vi "DOE Agilent Setup SUB.vi"(6 "Analog Channels-List":string, 7 "TC Type (K,J,T)":string, 8 "error in (no error)":errorcluster, 9 "TC Channels-List":string, 10 "Agilent Gain":dbl, 11 "VISA Refnum in":refnum<visa-resource-name>) -> (0 "error out":errorcluster, 2 "Clean Analog Scan List":string, 3 "Instrument IDN":string)   [LabVIEW 2016]
uses:
  Drivers/Agilent 34972/Agilent 34970.lvlib
panel:
  out "Total Clean Scan List":string
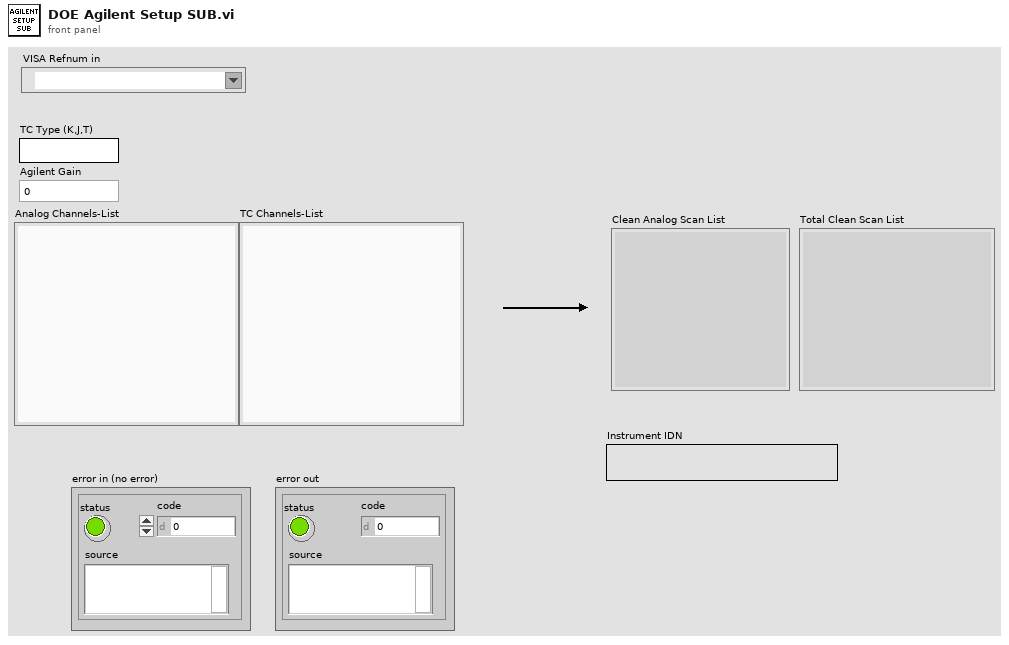
[diagram p1: front panel]
types:
  T1 = cluster{"Timeout Value (10000)":u32, "Baud Rate (57600)":enum16{"1200", "2400", "4800", "9600", "19200", "38400", "57600", "115200"}, "Flow Control (1:XON/XOFF)":enum16{"None", "XON / XOFF", "RTS / CTS", "DTR / DSR"}}
  T2 = enum16{"Thermocouple", "Thermistor", "RTD", "4-Wire RTD"}
  T3 = cluster{"Thermocouple Type (Last)":enum16{"B", "E", "J", "K", "N", "R", "S", "T", "Default (Last)"}, "TC Rjunction (2:Int)":enum16{"Fixed", "External", "Internal"}, "Fixed Rjunction Temp (0:Manual)":enum16{"Manual", "Minimum", "Maximum"}, "TC Auto Check? (F:Don't Check)":bool, "Rjunct Temp Value (0)":dbl}
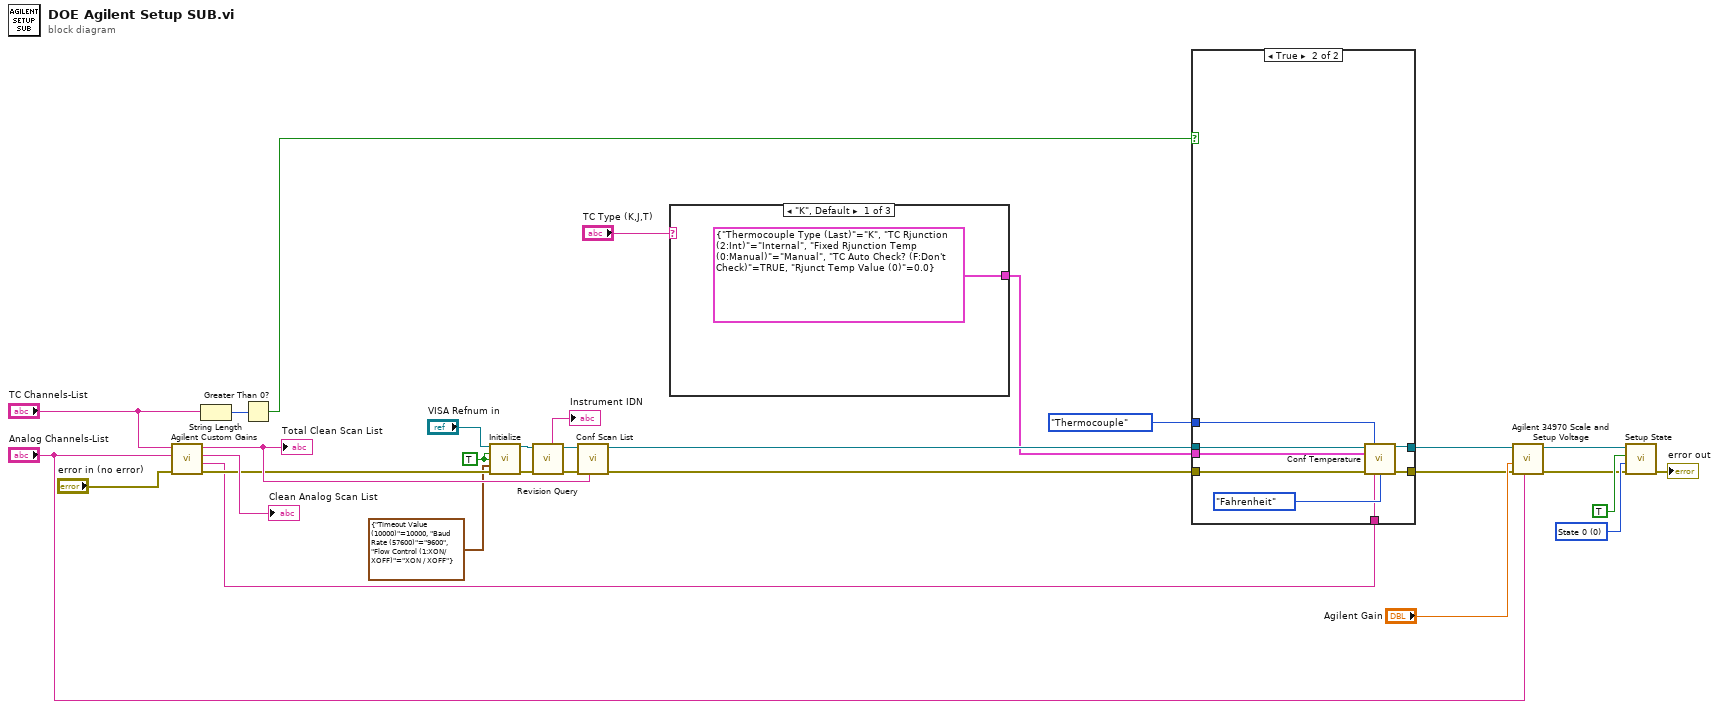
[diagram p0: block diagram]
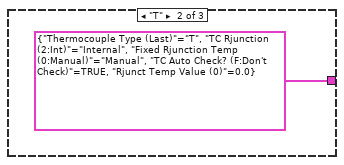
[diagram p3: hidden frame]
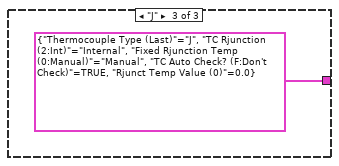
[diagram p4: hidden frame]
diagram:
  w11 = u16 0 items=["State 0", "State 1", "State 2", "State 3", "State 4", "State 5", "Preset State"] ("Setup State (6:Preset)")
  w26 = TRUE ("ID Query (T: Check)")
  n1 = call "Agilent Custom Gains.vi"("Error In"="error in (no error)", "Analog Channels-List"="Analog Channels-List", "TC Channels-List"="TC Channels-List") -> ("Error Out"=w3:errorcluster, "Clean TC Scan List"=w2:string, "Clean Analog Scan List"=→"Clean Analog Scan List":string, "Total Clean Scan List"=w12:string)  [unwired: 5 in]
  "Total Clean Scan List" <- w12
  n2 = String Length(string="TC Channels-List") -> (length=w15:i32)
  n3 = Greater Than 0?(x=w15) -> (x > 0?=w13:bool)
  n4 = call "Initialize.vi"("VISA Resource Name"="VISA Refnum in", "ID Query (T: Check)"=w26, "Reset (T: Reset)"=w26, "Serial Port Configuration"=T1 {"Timeout Value (10000)"=10000, "Baud Rate (57600)"=enum."9600", "Flow Control (1:XON/XOFF)"=enum."XON / XOFF"}, "error in (no error)"=w3) -> ("VISA Resource Name Out"=w25:refnum<visa-resource-name>, "error out"=w24:errorcluster)  [unwired: 9 in]
  n5 = call "Revision Query.vi"("error in (no error)"=w24, "VISA Resource Name"=w25) -> ("error out"=w23:errorcluster, "VISA Resource Name Out"=w22:refnum<visa-resource-name>, "Instrument IDN"=→"Instrument IDN":string)  [unwired: 5 in, 2 out]
  n6 = call "Conf Scan List.vi"("Scan List (empty)"=w12, "error in (no error)"=w23, "VISA Resource Name"=w22) -> ("error out"=w19:errorcluster, "VISA Resource Name Out"=w20:refnum<visa-resource-name>)  [unwired: 6 in, 1 out]
  n7 = case shown="\"K\", Default" "TC Type (K,J,T)" {
    tunnel: [T3 {"Thermocouple Type (Last)"=enum."K", "TC Rjunction (2:Int)"=enum."Internal", "Fixed Rjunction Temp (0:Manual)"=enum."Manual", "TC Auto Check? (F:Don't Check)"=TRUE, "Rjunct Temp Value (0)"=0.0} ("Thermocouple Configuration") T3 {"Thermocouple Type (Last)"=enum."T", "TC Rjunction (2:Int)"=enum."Internal", "Fixed Rjunction Temp (0:Manual)"=enum."Manual", "TC Auto Check? (F:Don't Check)"=TRUE, "Rjunct Temp Value (0)"=0.0} ("Thermocouple Configuration") T3 {"Thermocouple Type (Last)"=enum."J", "TC Rjunction (2:Int)"=enum."Internal", "Fixed Rjunction Temp (0:Manual)"=enum."Manual", "TC Auto Check? (F:Don't Check)"=TRUE, "Rjunct Temp Value (0)"=0.0} ("Thermocouple Configuration")] -> w16
    frame "K", Default {
    }
    frame "T" {
    }
    frame "J" {
    }
  }
  n8 = case shown="True" w13 {
    tunnel: T2."Thermocouple" ("Transducer Type (0:TC)") -> [_ w43]
    tunnel: w20 -> [w35 w41]
    tunnel: w19 -> [w34 w40]
    tunnel: [w34 w39] -> w18
    tunnel: [w35 w38] -> w17
    tunnel: w16 -> [_ w37]
    tunnel: w2 -> [_ w36]
    frame False {
    }
    frame True {
      n9 = call "Conf Temperature.vi"("VISA Resource Name"=w41, "Transducer Type (0:TC)"=w43, "Thermocouple Configuration"=w37, "error in (no error)"=w40, "Channel List(empty)"=w36, "Units (0:Celsius)"=enum16{"Celsius", "Fahrenheit", "Kelvin"}."Fahrenheit") -> ("VISA Resource Name Out"=w38:refnum<visa-resource-name>, "error out"=w39:errorcluster)  [unwired: 7 in, 1 out]
    }
  }
  n10 = call "Agilent 34970 Scale and Setup Voltage.vi"("Channel List"="Analog Channels-List", "error in (no error)"=w18, "Gain (1)"="Agilent Gain", "VISA Refnum in"=w17) -> ("error out"=w9:errorcluster, "VISA Refnum out"=w7:refnum<visa-resource-name>)  [unwired: 6 in]
  n11 = call "Setup State.vi"("error in (no error)"=w9, "Setup State (6:Preset)"=w11, "Recall/Save (F=Recall)"=TRUE, "VISA Resource Name"=w7) -> ("error out"=→"error out":errorcluster)  [unwired: 6 in, 1 out]
